vi "ReadingAttributes.vi"(0 "reference in":refnum<class "MyG#G3SubTempl.lvclass">, 5 "error in (no error)":errorcluster) -> (14 "reference out":refnum<class "MyG#G3SubTempl.lvclass">, 15 "Base class.MyAttribute":dbl, 16 "MySubAttribute":dbl, 19 "error out":errorcluster)   [LabVIEW 2017, in "MyG#G3SubTempl.lvclass"]
uses:
  MyG#G3SubTempl.lvclass
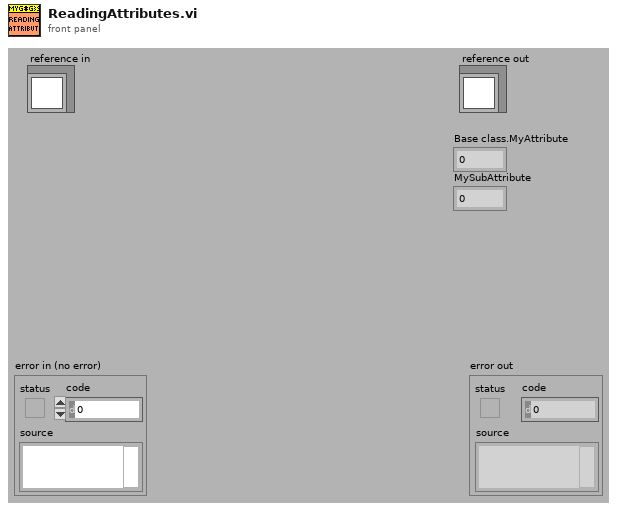
[diagram p1: front panel]
types:
  T1 = typedef "MyG#G3SubTempl.lvclass/ObjectAttributes.ctl" = cluster{"Base class":T2, "MySubAttribute":dbl}
  T2 = typedef "MyG#G3Templ.lvclass/ObjectAttributes.ctl" = cluster{"MyAttribute":dbl}
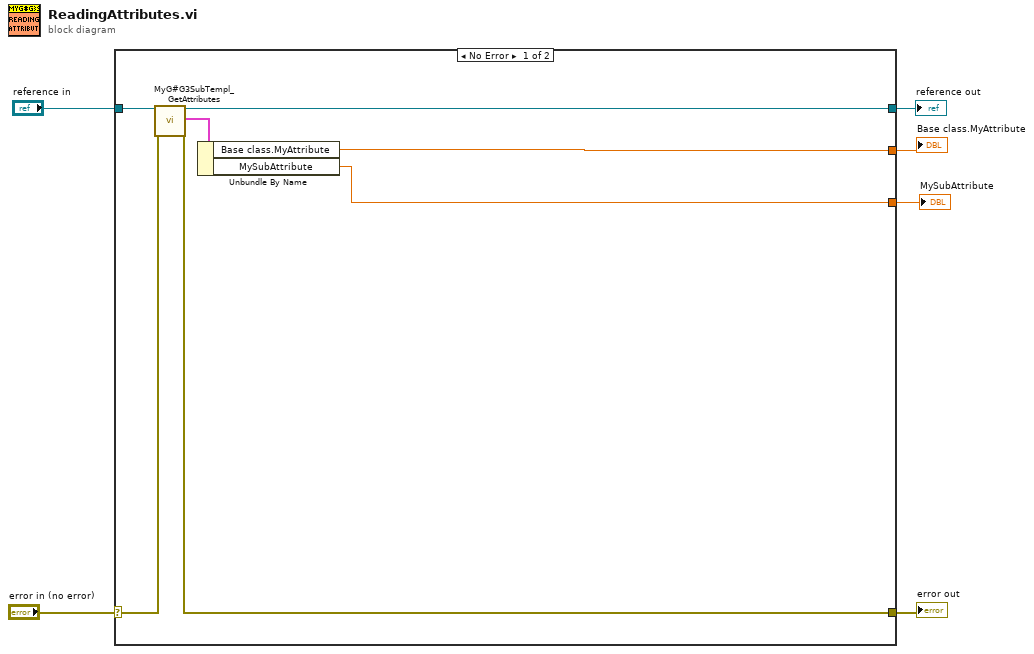
[diagram p0: block diagram]
diagram:
  n1 = case shown="No Error" "error in (no error)" {
    selector: "error in (no error)" -> [w13 w15]
    tunnel: [w11 w15] -> w5
    tunnel: [w9 w14] -> w3
    tunnel: "reference in" -> [w10 w14]
    tunnel: [w8 _] -> w2
    tunnel: [w7 _] -> w1
    frame No Error {
      n2 = call "MyG#G3SubTempl_GetAttributes.vi"("reference in"=w10, "error in (no error)"=w13) -> ("reference out"=w9:refnum<class "MyG#G3SubTempl.lvclass">, "attributes"=w12:T1, "error out"=w11:errorcluster)  [unwired: 14 in, 1 out]
      n3 = Unbundle By Name(w12) -> ("Base class.MyAttribute"=w8:dbl, "MySubAttribute"=w7:dbl)
    }
    frame Error {
    }
  }
  "error out" <- w5
  "reference out" <- w3
  "Base class.MyAttribute" <- w2
  "MySubAttribute" <- w1
